vi "Hardware_Module_z3.vi"(4 "Mode":enum16{"Normal", "Hidden"}(ring), 6 "Sine Wave":T1={"Frequency [Hz]"=50.0, "Amplitude [V]"=2.0, "Offset [V]"=2.5}, 7 "State":enum16{"Configure Port", "Read", "Close"}(ring), 8 "error in (no error)":errorcluster, 9 "byte count":u32, 10 "baud rate (9600)":u32=9600, 11 "VISA resource name":refnum<visa-resource-name>) -> (0 "error out":errorcluster, 2 "read buffer":string, 3 "VISA resource name out":refnum<visa-resource-name>)   [LabVIEW 2020]
doc: "Funkcja służy do komunikacji za pomocą portu szeregowergo z modułem EvB5.1, który zawiera mikroporcesor Atmega32. Komunikacja odbywa się poprzez bibliotekę NI-VISA z wykorzystaniem podstawowych funkcji portu szeregowego. Funkcja umożliwia emulację hardwaru i softwaru wówczas jako nazwę urządzenia podać: VirtualDevice1\n\n- VISA resource name specifies the resource to be opened.\n- baud rate is the rate of transmission. The default is 9600. \n- write buffer contains the data to be written to the device. \n- return count contains the actual number of bytes written. \n- State defines the functionality of the function. It contains three values Configure Port, Write and Close\n- LEDs is used during emulation. This is a reference to boolean array.\n- error out contains error information. This output provides standard error out functionality.\n\nWięcej pomocy można znaleźć w pomocy funkcji:\nVISA Configure Serial Port VI \nVISA Write Function"
uses:
  <vilib>/numeric/Random Number (Range) DBL.vi
  <vilib>/Instr/_visa.llb/VISA Configure Serial Port (Instr).vi
  <vilib>/measure/NI_MABase.lvlib
panel:
  # "Inputs"
  # "Outputs"
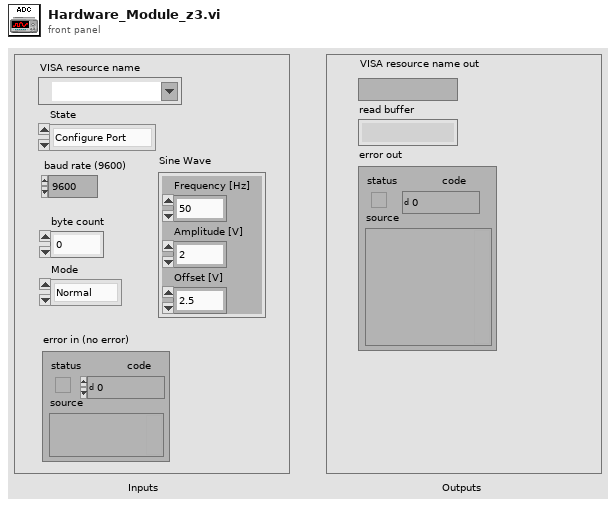
[diagram p1: front panel]
types:
  T1 = cluster{"Frequency [Hz]":dbl, "Amplitude [V]":dbl, "Offset [V]":dbl}
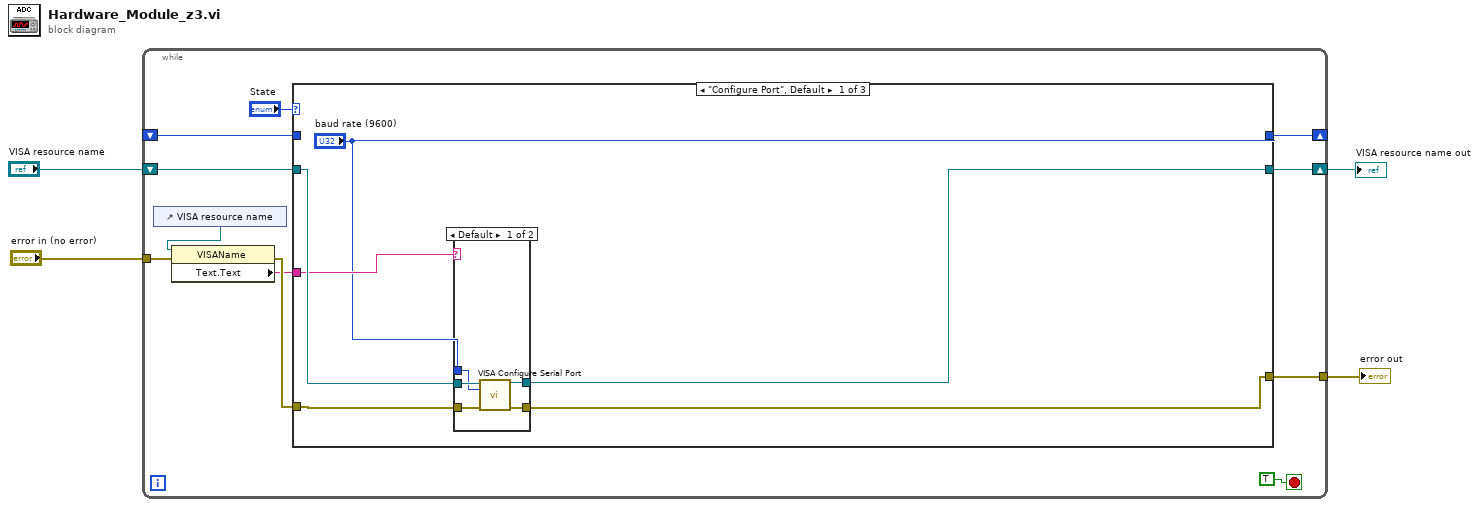
[diagram p0: block diagram]
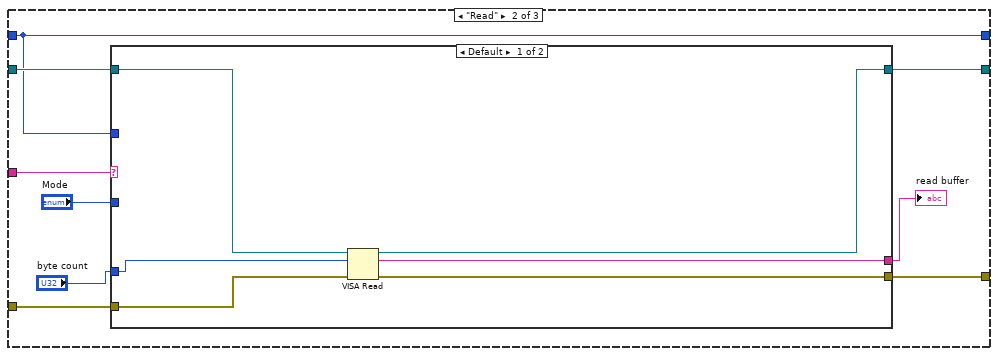
[diagram p3: hidden frame]
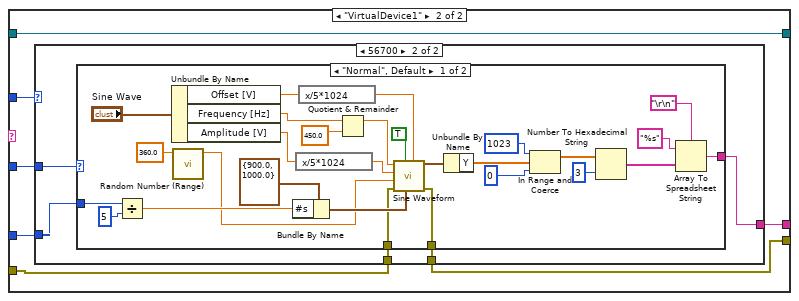
[diagram p4: hidden frame]
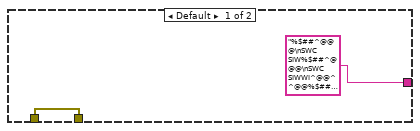
[diagram p5: hidden frame]
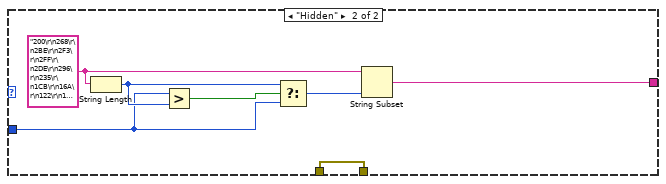
[diagram p6: hidden frame]
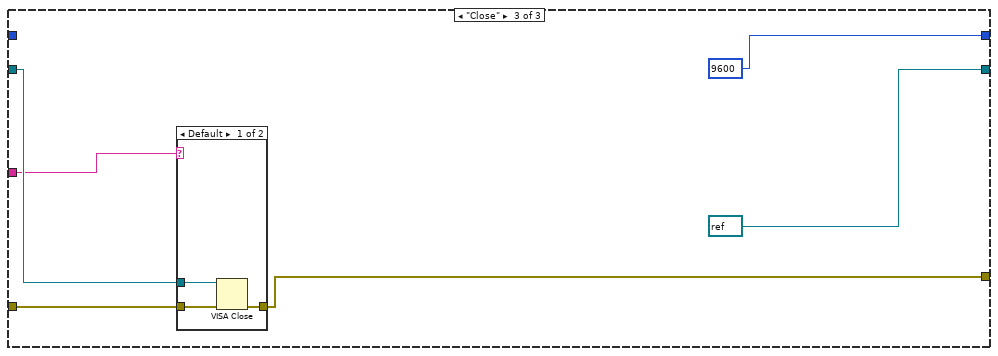
[diagram p7: hidden frame]
diagram:
  n1 = while {
    tunnel: "error in (no error)" -> [w14]
    tunnel: [w12] -> w2
    shift-right: [w13] -> w3
    shift-left: "VISA resource name" -> [w11]
    shift-right: [w9] -> _
    shift-left: _ -> [w6]
    stop <- TRUE stop-if-true
    n2 = control-ref of="VISA resource name"() -> (w5:refnum<vi>)
    n3 = property on="Property Node" class="VISAName"(reference=w5, error in=w14) -> (error out=w8:errorcluster, "Text.Text"=w7:string)  [unwired: 1 out]
    n4 = case shown="\"Configure Port\", Default" "State" {
      tunnel: [w21 w37 refnum<visa-resource-name> refnum ("VISA resource name")] -> w13
      tunnel: [w20 w32 w96] -> w12
      tunnel: w11 -> [w19 w36 w97]
      tunnel: ["baud rate (9600)" w31 u32 9600 ("baud rate (9600)")] -> w9
      tunnel: w8 -> [w18 w34 w94]
      tunnel: w7 -> [w17 w35 w95]
      tunnel: w6 -> [_ w31 _]
      frame "Configure Port", Default {
        n5 = case shown="Default" w17 {
          tunnel: w18 -> [w26 w28]
          tunnel: [w25 w27] -> w21
          tunnel: [w24 w28] -> w20
          tunnel: w19 -> [w23 w27]
          tunnel: "baud rate (9600)" -> [w22 _]
          frame Default {
            n6 = call-poly "VISA Configure Serial Port"("VISA resource name"=w23, "baud rate (9600)"=w22, "error in (no error)"=w26) -> ("VISA resource name out"=w25:refnum<visa-resource-name>, "error out"=w24:errorcluster)  [unwired: 11 in]
          }
          frame "VirtualDevice1" {
          }
        }
      }
      frame "Read" {
        n7 = case shown="Default" w35 {
          tunnel: w36 -> [w43 w50]
          tunnel: [w40 w44] -> w32
          tunnel: w34 -> [w41 w45]
          tunnel: [w42 w50] -> w37
          tunnel: [w39 w47] -> w33
          tunnel: w31 -> [_ w49]
          tunnel: "byte count" -> [w38 w48]
          tunnel: "Mode" -> [_ w46]
          frame Default {
            n8 = VISA Read(VISA resource name=w43, byte count=w38, error in (no error)=w41) -> (VISA resource name out=w42:refnum<visa-resource-name>, read buffer=w39:string, error out=w40:errorcluster)  [unwired: 1 out]
          }
          frame "VirtualDevice1" {
            n9 = case shown="56700" w49 {
              tunnel: w48 -> [_ w57]
              tunnel: ["%$##^@@@\nSWC SIW%$##^@@@\nSWC SIWWI^@@^^@@%$##^@@@\nSWC SIWWI^@@^^@@(!(!#!^#\n                     @!%@** JD  as1(!(!#!^#\n                     @!%@** JD  as1WI^@@^^@@(!(!#!^#\n                     @!%@** JD  as1" ("spreadsheet string") w56] -> w47
              tunnel: w46 -> [_ w55]
              tunnel: w45 -> [w51 w54]
              tunnel: [w51 w53] -> w44
              frame Default {
              }
              frame 56700 {
                n10 = case shown="\"Normal\", Default" w55 {
                  tunnel: w57 -> [w80 w88]
                  tunnel: [w76 w87] -> w56
                  tunnel: w54 -> [w64 w86]
                  tunnel: [w63 w86] -> w53
                  frame "Normal", Default {
                    n11 = Divide(x=w80, y=u32 5) -> (x/y=w79:dbl)
                    n12 = Unbundle By Name("Sine Wave") -> ("Offset [V]"=w72:dbl, "Frequency [Hz]"=w84:dbl, "Amplitude [V]"=w74:dbl)
                    n13 = call-poly <vilib>:"Random Number (Range).vi"("upper bound (100)"=360.0) -> ("number"=w59:dbl)  [unwired: 10 in]
                    n14 = Bundle By Name(cluster=cluster{"Fs":dbl, "#s":dbl} {"Fs"=900.0, "#s"=1000.0} ("sampling info"), "#s"=w79) -> (w81:cluster{"Fs":dbl, "#s":dbl})
                    n15 = expression code="x/5*1024"(w74) -> (w73:dbl)
                    n16 = expression code="x/5*1024"(w72) -> (w71:dbl)
                    n17 = Quotient & Remainder(x=w84, y=450.0) -> (x-y*floor(x/y)=w61:dbl)  [unwired: 1 out]
                    n18 = call <vilib>:"Sine Waveform.vi"("offset"=w71, "sampling info"=w81, "reset signal"=TRUE, "error in (no error)"=w64, "phase"=w59, "amplitude"=w73, "frequency"=w61) -> ("error out"=w63:errorcluster, "signal out"=w78:waveform(dbl))  [unwired: 3 in]
                    n19 = Unbundle By Name(w78) -> ("Y"=w65:dbl[])
                    n20 = In Range and Coerce(upper limit=i16 1023 ("width (-)"), x=w65, lower limit=i16 0 ("width (-)")) -> (coerced(x)=w67:dbl[])  [unwired: 1 out]
                    n21 = Number To Hexadecimal String(1:i16 3 ("width (-)"), 2:w67) -> (0:w66:string[])
                    n22 = Array To Spreadsheet String(delimiter (Tab)="\r\n", array=w66, 3:"%s" ("format string")) -> (spreadsheet string=w76:string)
                  }
                  frame "Hidden" {
                    w89 = "200\r\n268\r\n2BE\r\n2F3\r\n2FF\r\n2DE\r\n296\r\n235\r\n1CB\r\n16A\r\n122\r\n101\r\n10D\r\n142\r\n198\r\n200\r\n268\r\n2BE\r\n2F3\r\n2FF\r\n2DE\r\n296\r\n235\r\n1CB\r\n16A\r\n122\r\n101\r\n10D\r\n142\r\n198\r\n200\r\n268\r\n2BE\r\n2F3\r\n2FF\r\n2DE\r\n296\r\n235\r\n1CB\r\n16A\r\n122\r\n101\r\n10D\r\n142\r\n198\r\n200\r\n268\r\n2BE\r\n2F3\r\n2FF\r\n2DE\r\n296\r\n235\r\n1CB\r\n16A\r\n122\r\n101\r\n10D\r\n142\r\n198\r\n200\r\n268\r\n2BE\r\n2F3\r\n2FF\r\n2DE\r\n296\r\n235\r\n1CB\r\n16A\r\n122\r\n101\r\n10D\r\n142\r\n198\r\n200\r\n268\r\n2BE\r\n2F3\r\n2FF\r\n2DE\r\n296\r\n235\r\n1CB\r\n16A\r\n122\r\n101\r\n10D\r\n142\r\n198\r\n200\r\n268\r\n2BE\r\n2F3\r\n2FF\r\n2DE\r\n296\r\n235\r\n1CB\r\n16A\r\n122\r\n101\r\n10D\r\n142\r\n198\r\n200\r\n268\r\n2BE\r\n2F3\r\n2FF\r\n2DE\r\n296\r\n235\r\n1CB\r\n16A\r\n122\r\n101\r\n10D\r\n142\r\n198\r\n..." ("spreadsheet string")
                    n23 = String Length(string=w89) -> (length=w92:i32)
                    n24 = Greater?(x=w88, y=w92) -> (0:w90:bool)
                    n25 = Select(t=w92, s=w90, f=w88) -> (s? t:f=w91:u32)
                    n26 = String Subset(string=w89, length (rest)=w91) -> (substring=w87:string)  [unwired: 1 in]
                  }
                }
              }
            }
          }
        }
        "read buffer" <- w33
      }
      frame "Close" {
        n27 = case shown="Default" w95 {
          tunnel: w97 -> [w101 _]
          tunnel: [w100 w102] -> w96
          tunnel: w94 -> [w99 w102]
          frame Default {
            n28 = VISA Close(VISA resource name=w101, error in (no error)=w99) -> (error out=w100:errorcluster)
          }
          frame "VirtualDevice1" {
          }
        }
      }
    }
  }
  "VISA resource name out" <- w3
  "error out" <- w2
